vi "Lock or Unlock Front Panel.vi"(7 "Unit ID (A)":string="A", 8 "error in":errorcluster, 10 "Lock/Unlock":enum8{"Unlock", "Lock"}(ring), 11 "VISA Session In":refnum<visa-resource-name>="Alicat") -> (0 "error out":errorcluster, 3 "VISA Session Out":refnum<visa-resource-name>)   [LabVIEW 2015]
doc: "Locks or unlocks the front panel. A locked Alicat front panel will not allow users to make any changes using the push button menu."
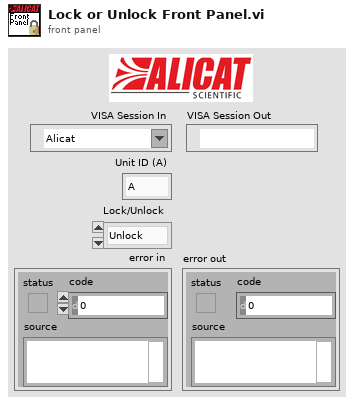
[diagram p1: front panel]
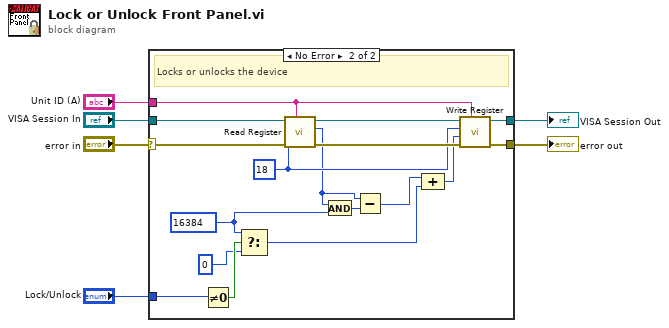
[diagram p0: block diagram]
diagram:
  n1 = case shown="No Error" "error in" {
    selector: "error in" -> [w7 w25]
    tunnel: "VISA Session In" -> [w8 w24]
    tunnel: [w7 w13] -> w4
    tunnel: [w8 w22] -> w3
    tunnel: "Unit ID (A)" -> [_ w20]
    tunnel: "Lock/Unlock" -> [_ w11]
    frame Error {
    }
    frame No Error {
      w10 = 16384 ("y")
      w14 = u16 18 ("register")
      # "Locks or unlocks the device"
      n2 = Not Equal To 0?(x=w11) -> (x != 0?=w18:bool)
      n3 = Select(t=w10, s=w18, f=0 ("y")) -> (s? t:f=w9:i32)
      n4 = call "Read Register.vi"("Unit ID (A)"=w20, "error in"=w25, "Register address"=w14, "VISA Session In"=w24) -> ("error out"=w23:errorcluster, "Register Value (I32)"=w12:i32, "VISA Session Out"=w21:refnum<visa-resource-name>)  [unwired: 5 in]
      n5 = And(x=w12, y=w10) -> (x .and. y?=w19:i32)
      n6 = Subtract(x=w12, y=w19) -> (x-y=w16:i32)
      n7 = Compound Arithmetic op=ADD(w16, w9) -> (w15:i32)
      n8 = call "Write Register.vi"("Unit ID (A)"=w20, "error in"=w23, "Register Value"=w15, "Register address"=w14, "VISA Session In"=w21) -> ("error out"=w13:errorcluster, "VISA Session Out"=w22:refnum<visa-resource-name>)  [unwired: 4 in, 1 out]
    }
  }
  "error out" <- w4
  "VISA Session Out" <- w3
